vi "Create Connection.vi"(8 "error in (no error)":errorcluster, 11 "ConnectionFactoryHandler in":refnum<class "ConnectionFactoryHandler.lvclass">) -> (0 "error out":errorcluster, 3 "ConnectionFactoryHandler out":refnum<class "ConnectionFactoryHandler.lvclass">)   [LabVIEW 2020, in "ConnectionFactorySession.lvlib" / "ConnectionFactoryHandler.lvclass"]
uses:
  <vilib>/gpm_packages/@cs/Network-interface/Source/Connection Factory Session/ConnectionFactoryHandler/ConnectionFactoryHandler.lvclass
  C:/Program Files/National Instruments/LabVIEW 2020/vi.lib/gpm_packages/@cs/Network-interface/Source/Logged Actor/LoggedActor.lvclass
  C:/Program Files/National Instruments/LabVIEW 2020/vi.lib/ActorFramework/Actor/Actor.lvclass
  <vilib>/gpm_packages/@cs/Network-interface/Source/Connection Reference/IConnection/IConnection.lvclass
  <vilib>/gpm_packages/@cs/Network-interface/Source/Connection Factory Session/ConnectionFactoryHandler/ConnectionFactoryHandler.lvclass/ConnectionFactoryHandler.ctl
  <vilib>/gpm_packages/@cs/event-logger/Source/Composed Log/Types/Log Level.ctl
  <vilib>/gpm_packages/@cs/Network-interface/Source/Logged Actor/LoggedActor.lvclass/LoggedActor.ctl
  <vilib>/gpm_packages/@cs/event-logger/Source/Composed Log/LoggerReference/LoggerReference.lvclass/LoggerReference.ctl
  <vilib>/ActorFramework/Actor/Actor.lvclass/Actor.ctl
  <vilib>/ActorFramework/Message Enqueuer/Message Enqueuer.lvclass/Message Enqueuer.ctl
  <vilib>/ActorFramework/Message Enqueuer/Enqueue.vi
  <vilib>/ActorFramework/Message Enqueuer/Init from Existing Queue.vi
  <vilib>/gpm_packages/@cs/event-logger/Source/Composed Log/LoggerReference/Log Event.vi
  <vilib>/gpm_packages/@cs/event-logger/Source/Composed Log/LoggerReference/Log.vi
  <vilib>/gpm_packages/@cs/event-logger/Source/Composed Log/LoggerReference/Get Valid Event Time.vi
  <vilib>/gpm_packages/@cs/event-logger/Source/Composed Log/LoggerReference/Remove Stale Logs.vi
  <vilib>/gpm_packages/@cs/Network-interface/Source/Connection Factory Session/Messages/Create Connection Msg/Create Connection Msg.lvclass
  C:/Program Files/National Instruments/LabVIEW 2020/vi.lib/ActorFramework/Message/Message.lvclass
  <vilib>/ActorFramework/Message Priority Queue/Priority Enqueue.vi
  <vilib>/gpm_packages/@cs/Network-interface/Source/Connection Reference/Connection Reference/Connection Reference.lvclass
  <vilib>/ActorFramework/Message Enqueuer/Message Enqueuer.lvclass
  <vilib>/gpm_packages/@cs/Network-interface/Source/IConnectionFactory/IConnectionFactory.lvclass
  <vilib>/gpm_packages/@cs/Network-interface/Source/Connection Factory Session/INewConnectionCallback/INewConnectionCallback.lvclass
  <vilib>/ActorFramework/Actor/Actor.lvclass
  <vilib>/gpm_packages/@cs/Network-interface/Source/Logged Actor/LoggedActor.lvclass
  <vilib>/gpm_packages/@cs/event-logger/Source/Composed Log/Composed Log.lvlib
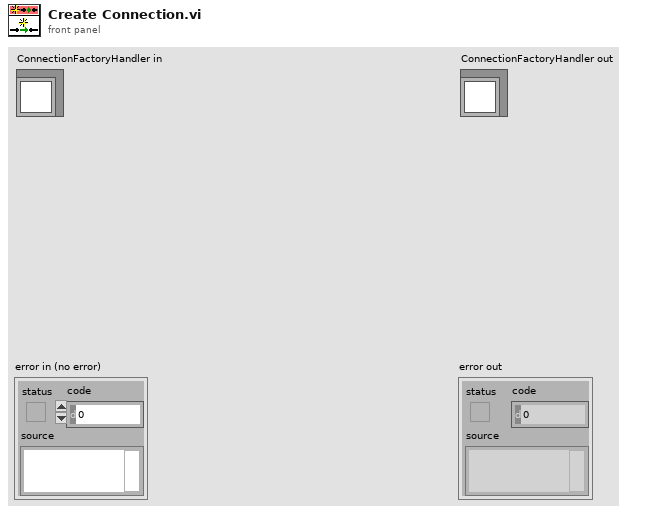
[diagram p1: front panel]
types:
  T1 = typedef "Composed Log.lvlib/Log Level.ctl" = enum16{"Debug", "Info", "Warning", "Error", "Critical"}
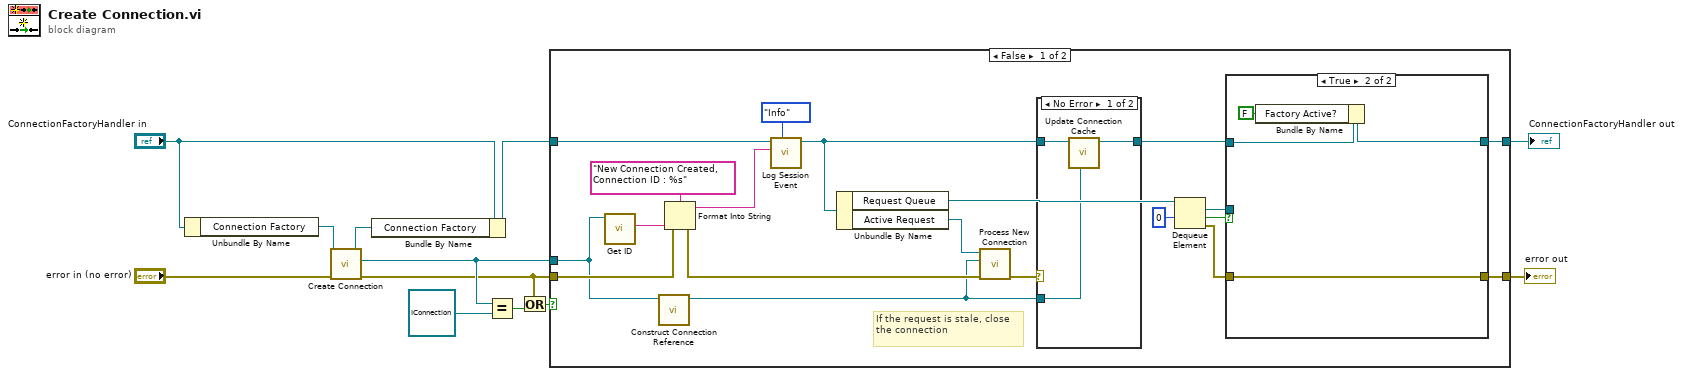
[diagram p0: block diagram]
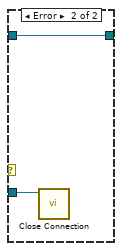
[diagram p2: hidden frame]
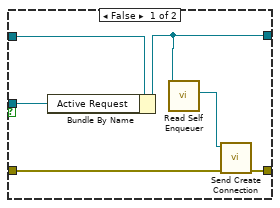
[diagram p3: hidden frame]
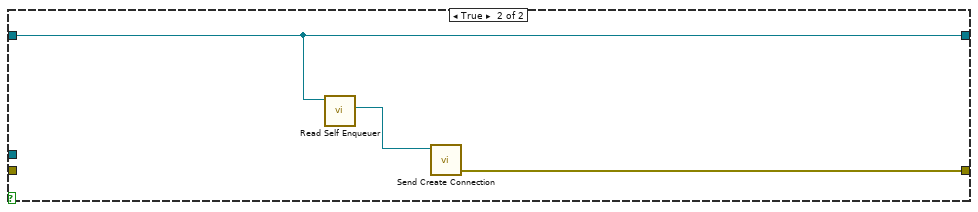
[diagram p4: hidden frame]
diagram:
  n1 = Unbundle By Name("ConnectionFactoryHandler in") -> ("Connection Factory"=w12:refnum<class "IConnectionFactory.lvclass">)
  n2 = call-dynamic "Create Connection.vi"("error in (no error)"="error in (no error)", "IConnectionFactory in"=w12) -> ("error out"=w3:errorcluster, "Connection"=w6:refnum<class "IConnection.lvclass">, "IConnectionFactory out"=w11:refnum<class "IConnectionFactory.lvclass">)  [unwired: 7 in]
  n3 = Bundle By Name(cluster="ConnectionFactoryHandler in", "Connection Factory"=w11) -> (w8:refnum<class "ConnectionFactoryHandler.lvclass">)
  n4 = Equal?(x=w6, y=refnum<class "IConnection.lvclass"> refnum) -> (x = y?=w2:bool)
  n5 = Or(x=w3, y=w2) -> (x .or. y?=w1:bool)
  n6 = case shown="False" w1 {
    tunnel: w6 -> [w16 _]
    tunnel: w8 -> [w24 w50]
    tunnel: [w32 w50] -> w7
    tunnel: w3 -> [w19 _]
    tunnel: [w26 w48] -> w4
    frame False {
      # "If the request is stale, close the connection"
      n7 = call-dynamic "Get ID.vi"("IConnection in"=w16) -> ("ID"=w22:string)  [unwired: 10 in]
      n8 = call <vilib>:"Construct Connection Reference.vi"("Connection"=w16) -> ("Connection Reference"=w15:refnum<data-value>)  [unwired: 9 in, 1 out]
      n9 = Format Into String(format string="New Connection Created, Connection ID : %s", error in=w19, w22) -> (resulting string=w20:string, error out=w18:errorcluster)  [unwired: 1 in]
      n10 = call <vilib>:"Log Session Event.vi"("Event Level"=Log_Level."Info", "Event Data"=w20, "SessionActor in"=w24) -> ("SessionActor out"=w14:refnum<class "ConnectionFactoryHandler.lvclass">)  [unwired: 7 in, 1 out]
      n11 = Unbundle By Name(w14) -> ("Request Queue"=w30:refnum<queue>, "Active Request"=w31:refnum<class "INewConnectionCallback.lvclass">)
      n12 = call-dynamic "Process New Connection.vi"("error in (no error)"=w18, "New Connection Reference"=w15, "INewConnectionCallback in"=w31) -> ("error out"=w17:errorcluster)  [unwired: 8 in]
      n13 = case shown="No Error" w17 {
        tunnel: w15 -> [w33 w37]
        tunnel: w14 -> [w35 w36]
        tunnel: [w34 w36] -> w13
        frame No Error {
          n14 = call <vilib>:"Update Connection Cache.vi"("Connection Reference"=w33, "ConnectionFactoryHandler in"=w35) -> ("ConnectionFactoryHandler out"=w34:refnum<class "ConnectionFactoryHandler.lvclass">)  [unwired: 9 in]
        }
        frame Error {
          n15 = call <vilib>:"Close Connection.vi"("Connection Reference In"=w37) -> ()  [unwired: 10 in, 1 out]
        }
      }
      n16 = Dequeue Element(queue=w30, timeout in ms (-1)=0) -> (element=w28:refnum<class "INewConnectionCallback.lvclass">, timed out?=w27:bool, error out=w25:errorcluster)  [unwired: 1 in, 1 out]
      n17 = case shown="True" w27 {
        tunnel: w13 -> [w43 w47]
        tunnel: [w41 w46] -> w32
        tunnel: w28 -> [w42 _]
        tunnel: w25 -> [w40 w44]
        tunnel: [w39 w44] -> w26
        frame False {
          n18 = Bundle By Name(cluster=w43, "Active Request"=w42) -> (w41:refnum<class "ConnectionFactoryHandler.lvclass">)
          n19 = call <vilib>:"Read Self Enqueuer.vi"("Actor"=w41) -> ("Self Enqueuer"=w38:refnum<class "Message Enqueuer.lvclass">)  [unwired: 10 in]
          n20 = call <vilib>:"Send Create Connection.vi"("error in (no error)"=w40, "Message Enqueuer"=w38) -> ("error out"=w39:errorcluster)  [unwired: 8 in, 1 out]
        }
        frame True {
          n21 = Bundle By Name(cluster=w47, "Factory Active?"=FALSE) -> (w46:refnum<class "ConnectionFactoryHandler.lvclass">)
        }
      }
    }
    frame True {
      n22 = call <vilib>:"Read Self Enqueuer.vi"("Actor"=w50) -> ("Self Enqueuer"=w49:refnum<class "Message Enqueuer.lvclass">)  [unwired: 10 in]
      n23 = call <vilib>:"Send Create Connection.vi"("Message Enqueuer"=w49) -> ("error out"=w48:errorcluster)  [unwired: 9 in, 1 out]
    }
  }
  "error out" <- w4
  "ConnectionFactoryHandler out" <- w7
